vi "Get Data Type Name.vi"(11 "String Type View in":refnum<class "String Type View.lvclass">) -> (3 "Data Type Name":string="Default Data Type")   [LabVIEW 2017, in "String Type View.lvclass"]
uses:
  <vilib>/gpm_packages/@cs/Test-executive-builder/Source/Test Executive Builder Dialogs/String Type View/String Type View.lvclass
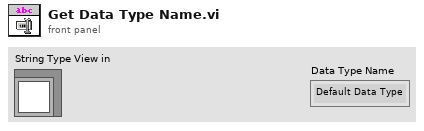
[diagram p1: front panel]
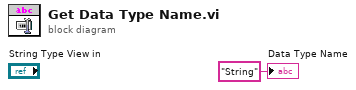
[diagram p0: block diagram]
diagram:
  "Data Type Name" <- "String" ("Data Type Name")
